vi "Auto Homing.vi"() -> (2 "Turret Angle to go to 2":dbl(slide) scale=-180.0..180.0)   [LabVIEW 2019]
uses:
  Framework/Robot Global Data.vi
panel:
  out "Turret Angle to go to":dbl
  out "Final Turret Angle":dbl
  out "Final Angle":dbl(slide) scale=-180.0..180.0
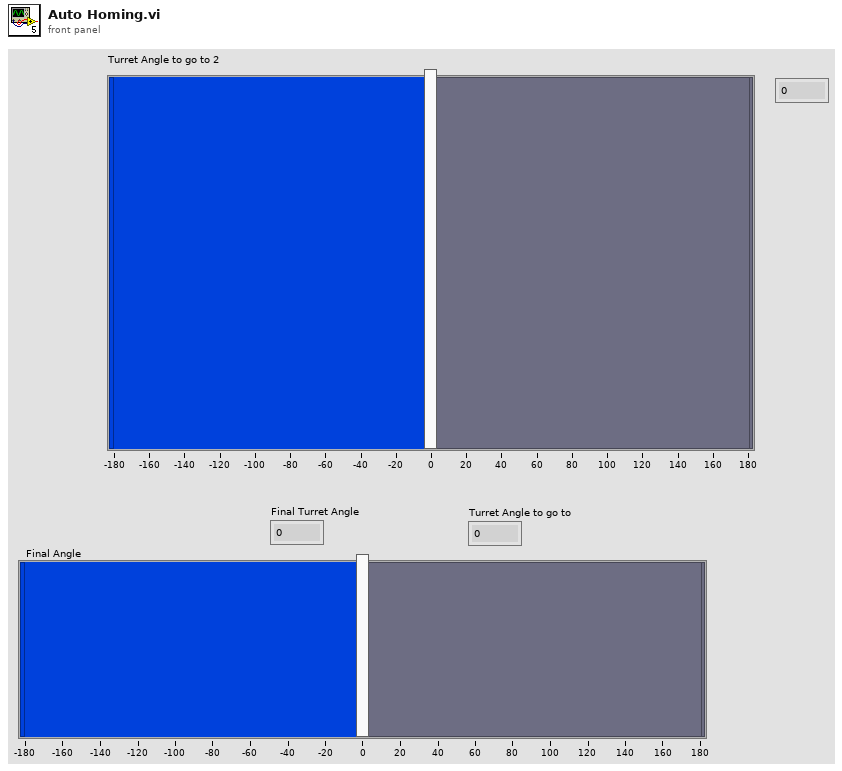
[diagram p1: front panel]
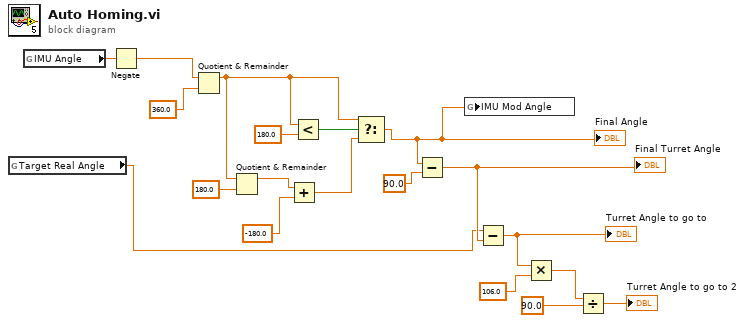
[diagram p0: block diagram]
diagram:
  n1 = global read "Robot Global Data.vi" "Target Real Angle"() -> (w2:dbl)
  n2 = global read "Robot Global Data.vi" "IMU Angle"() -> (w18:dbl)
  n3 = Negate(x=w18) -> (-x=w17:dbl)
  n4 = Quotient & Remainder(x=w17, y=360.0) -> (x-y*floor(x/y)=w3:dbl)  [unwired: 1 out]
  n5 = Quotient & Remainder(x=w3, y=180.0) -> (x-y*floor(x/y)=w12:dbl)  [unwired: 1 out]
  n6 = Add(x=w12, y=-180.0) -> (x+y=w11:dbl)
  n7 = Less?(x=w3, y=180.0) -> (x < y?=w15:bool)
  n8 = Select(t=w3, s=w15, f=w11) -> (s? t:f=w1:dbl)
  "Final Angle" <- w1
  n9 = Subtract(x=w1, y=90.0) -> (x-y=w9:dbl)
  "Final Turret Angle" <- w9
  n10 = global write "Robot Global Data.vi" "IMU Mod Angle"(w1) -> ()
  n11 = Subtract(x=w2, y=w9) -> (x-y=w8:dbl)
  "Turret Angle to go to" <- w8
  n12 = Multiply(x=w8, y=106.0) -> (x*y=w6:dbl)
  n13 = Divide(x=w6, y=90.0) -> (x/y=→"Turret Angle to go to 2":dbl)
